vi "Data Client.vi"() -> ()   [LabVIEW 2011]
doc: "Displays data sent via TCP from Data Server.vi. Once a TCP connection is open, the VI reads 4 bytes to determine the amount of data being sent. It then reads and charts that many bytes. If an error occurs or the stop button is pressed, it sends a \"Q\" to the Data Sender to notify it to quit.\n\n<B>Note:</B> Requires the Data Server.vi located in the same library as this VI."
panel:
  out "data 3":sgl
  out "data 4":i32
  out "data 2":sgl
  out "data1":sgl
  in  "stop":bool
  out "chart":dbl[](graph)
  in  "Address":string="localhost"
  in  "Port":u16=6340 min=1025 step=1
  # "Instructions:\n1. Open the Data Server.vi located in the same library.\n2. Follow the instructions on it's front panel.\n\nNote: This VI is built to work with the Data Server.vi."
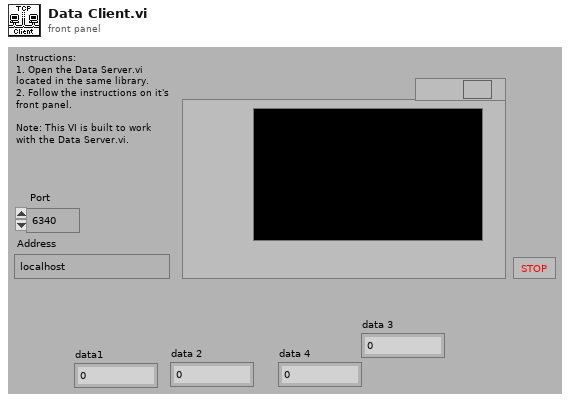
[diagram p1: front panel]
types:
  T1 = enum16{"Standard", "Buffered", "CRLF", "Immediate"}
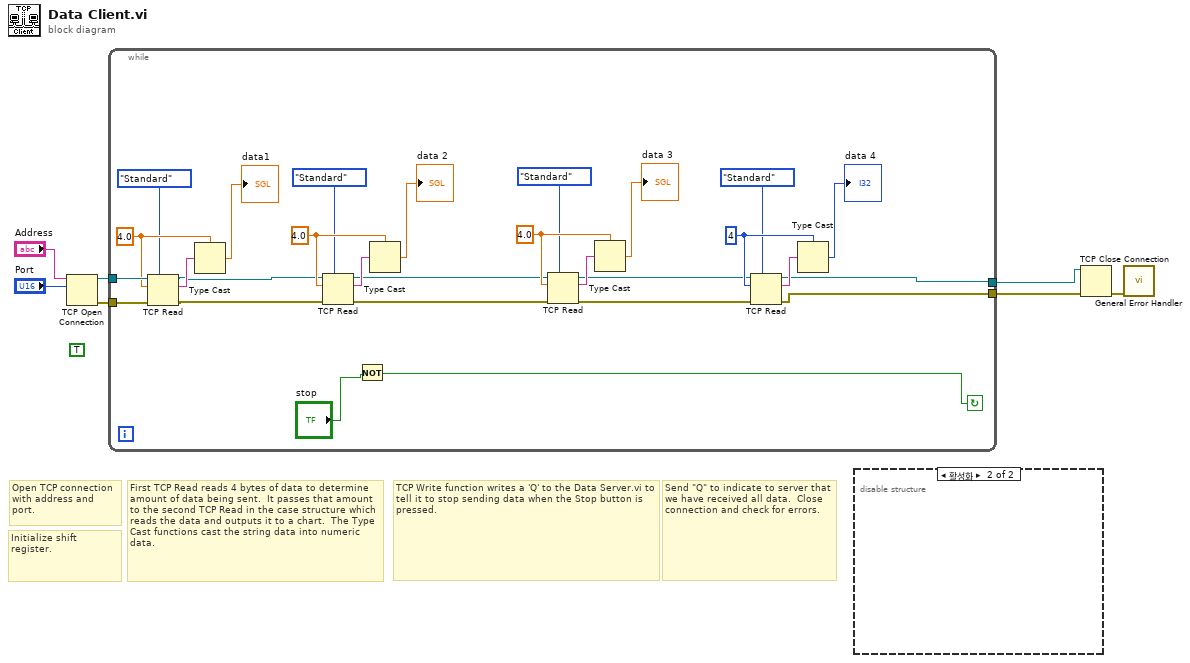
[diagram p0: block diagram]
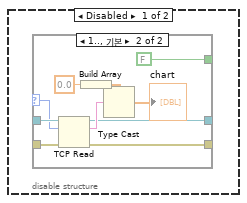
[diagram p2: hidden frame]
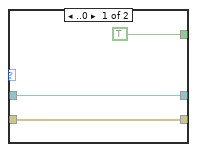
[diagram p3: hidden frame]
diagram:
  (unwired) TRUE
  # "Send \"Q\" to indicate to server that we have received all data.  Close connection and check for errors."
  # "TCP Write function writes a 'Q' to the Data Server.vi to tell it to stop sending data when the Stop button is pressed."
  # "First TCP Read reads 4 bytes of data to determine amount of data being sent.  It passes that amount to the second TCP Read in the case structure which reads the data and outputs it to a chart.  The Type Cast functions cast the string data into numeric data."
  # "Initialize shift register."
  # "Open TCP connection with address and port."
  n1 = TCP Open Connection(address="Address", remote port or service name="Port") -> (connection ID=w4:refnum<k5>, error out=w3:errorcluster)  [unwired: 1 in, 2 out]
  n2 = while {
    tunnel: w3 -> [w31]
    tunnel: w4 -> [w32]
    tunnel: [w16] -> w2
    tunnel: [w13] -> w1
    stop <- w14 continue-if-true
    w11 = sgl 4.0
    w20 = 4
    w26 = sgl 4.0
    w30 = sgl 4.0
    n3 = TCP Read(connection ID=w32, bytes to read=w30, error in (no error)=w31, 7:T1."Standard" ("모드(standard)")) -> (connection ID out=w23:refnum<k5>, data out=w33:string, error out=w22:errorcluster)  [unwired: 1 out]
    n4 = Type Cast(type=w30, x=w33) -> (*(type *) &x=→"data1":sgl)
    n5 = TCP Read(connection ID=w23, bytes to read=w26, error in (no error)=w22, 7:T1."Standard" ("모드(standard)")) -> (connection ID out=w8:refnum<k5>, data out=w27:string, error out=w17:errorcluster)  [unwired: 1 out]
    n6 = Not(x="stop") -> (.not. x?=w14:bool)
    n7 = Type Cast(type=w26, x=w27) -> (*(type *) &x=→"data 2":sgl)
    n8 = TCP Read(bytes to read=w11, 7:T1."Standard" ("모드(standard)")) -> (data out=w12:string)  [unwired: 2 in, 3 out]
    n9 = Type Cast(type=w11, x=w12) -> (*(type *) &x=→"data 3":sgl)
    n10 = TCP Read(connection ID=w8, bytes to read=w20, error in (no error)=w17, 7:T1."Standard" ("모드(standard)")) -> (connection ID out=w16:refnum<k5>, data out=w21:string, error out=w13:errorcluster)  [unwired: 1 out]
    n11 = Type Cast(type=w20, x=w21) -> (*(type *) &x=→"data 4":i32)
  }
  n12 = disable-structure shown="활성화" {
    frame Disabled {
      n13 = case shown="1.., 기본" {
        selector: _ -> [_ w41]
        tunnel: _ -> [w34 w44]
        tunnel: _ -> [w36 w43]
        tunnel: [w36 w42] -> _
        tunnel: [TRUE FALSE] -> _
        tunnel: [w34 w39] -> _
        frame ..0 {
        }
        frame 1.., Default {
          n14 = TCP Read(connection ID=w43, bytes to read=w41, error in (no error)=w44) -> (connection ID out=w42:refnum<k5>, data out=w45:string, error out=w39:errorcluster)  [unwired: 2 out]
          n15 = Build Array(0.0) -> (w37:dbl[])
          n16 = Type Cast(type=w37, x=w45) -> (*(type *) &x=→"chart":dbl[])
        }
      }
    }
    frame Enabled {
    }
  }
  n17 = TCP Close Connection(connection ID=w2, error in (no error)=w1) -> (error out=w5:errorcluster)  [unwired: 2 out]
  n18 = call <vilib>:"General Error Handler.vi"("error in (no error)"=w5) -> ()  [unwired: 1 in, 14 out]
